vi "Polish Control.vi"(10 "Control Ref":refnum<vi>, 11 "Number Writer in":refnum<class "Number Writer.lvclass">) -> (3 "Number Writer out":refnum<class "Number Writer.lvclass">)   [LabVIEW 2013, in "Number Writer.lvclass"]
doc: "Copyright (c) 2016 Sze Howe Koh\n\nThis Source Code Form is subject to the terms of the Mozilla Public License, v. 2.0. If a copy of the MPL was not distributed with this file, You can obtain one at http://mozilla.org/MPL/2.0/."
uses:
  Number Writer.lvclass
  Number Writer.lvclass/Number Writer.ctl
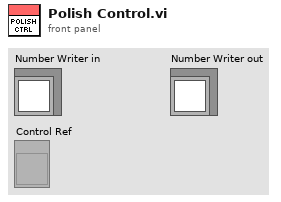
[diagram p1: front panel]
types:
  T1 = typedef "Number Writer.lvclass/Numeric Type.ctl" = enum16{"I8", "I16", "I32", "I64", "U8", "U16", "U32", "U64", "SGL", "DBL", "PTR INT", "PTR UINT"}
  T2 = typedef "LVNumericRepresentation.ctl" = enum32{"Extended Precision", "Double Precision", "Single Precision", "Long", "Word", "Byte", "Unsigned Long", "Unsigned Word", "Unsigned Byte", "Complex Extended", "Complex Double", "Complex Single", "Quad", "Unsigned Quad", "Fixed-Point"}
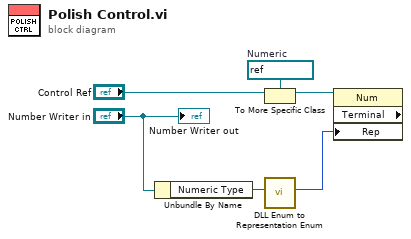
[diagram p0: block diagram]
diagram:
  w4 = refnum<vi> refnum  # Numeric
  n1 = Unbundle By Name("Number Writer in") -> ("Numeric Type"=w3:T1)
  n2 = To More Specific Class(target class=w4, reference="Control Ref") -> (specific class reference=w6:refnum<vi>)  [unwired: 1 in, 1 out]
  n3 = call "DLL Enum to Representation Enum.vi"("Numeric Type"=w3) -> ("Representation"=w5:T2)  [unwired: 10 in]
  n4 = property class="Num" props=["Terminal", "Rep"](reference=w6, "Rep"=w5) -> ()  [unwired: 1 in, 3 out]
  "Number Writer out" <- "Number Writer in"
